vi "TeledyneVueCommand.vi"(4 "Channel Name":string="TeleVue:Mdot:Meas(g/min)", 6 "Port Name":string="tcp://192.168.124.71:10001", 7 "Timeout/ms":u32=1500, 8 "Numeric Value":dbl format="%.6g", 9 "TeledyneVueCommand":T2="FullScaleRatingSLPM", 10 "Address":u8=186 format="%.0x") -> (0 "String Reply":string="!11,100.0000\r\n", 1 "Error Description":string, 2 "Numeric Reply":dbl=100.0 format="%_6g", 3 "OK":bool)   [LabVIEW 2017]
uses:
  TeledyneVueCommand.ctl
  TeledyneDFCCommandDescriptor.ctl
  TeledyneVueCommandPhases.ctl
panel:
  out "commandString":string
  out "Audit trail":string[](array[string])
  out "CommandDescriptorOutput":T1={"Command"="FullScaleRatingSLPM", "Mnemonic"="E", "Min"=nan, "Max"=nan, "ActionPath"=["PassCommand", "Communicate", "ParseNumber", "Done"]}
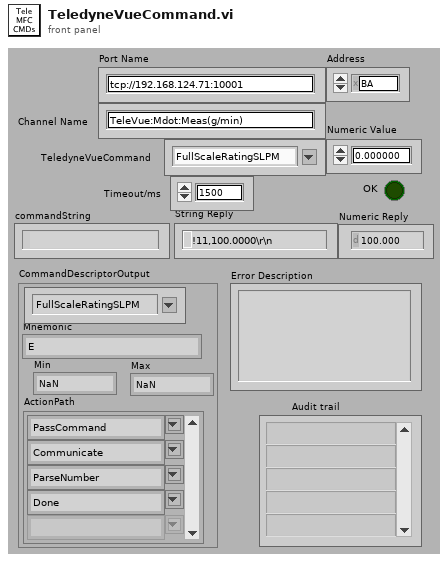
[diagram p1: front panel]
types:
  T1 = typedef "TeledyneDFCCommandDescriptor.ctl" = cluster{"Command":T2, "Mnemonic":string, "Min":dbl, "Max":dbl, "ActionPath":T3[]}
  T2 = typedef "TeledyneVueCommand.ctl" = string
  T3 = typedef "TeledyneVueCommandPhases.ctl" = string
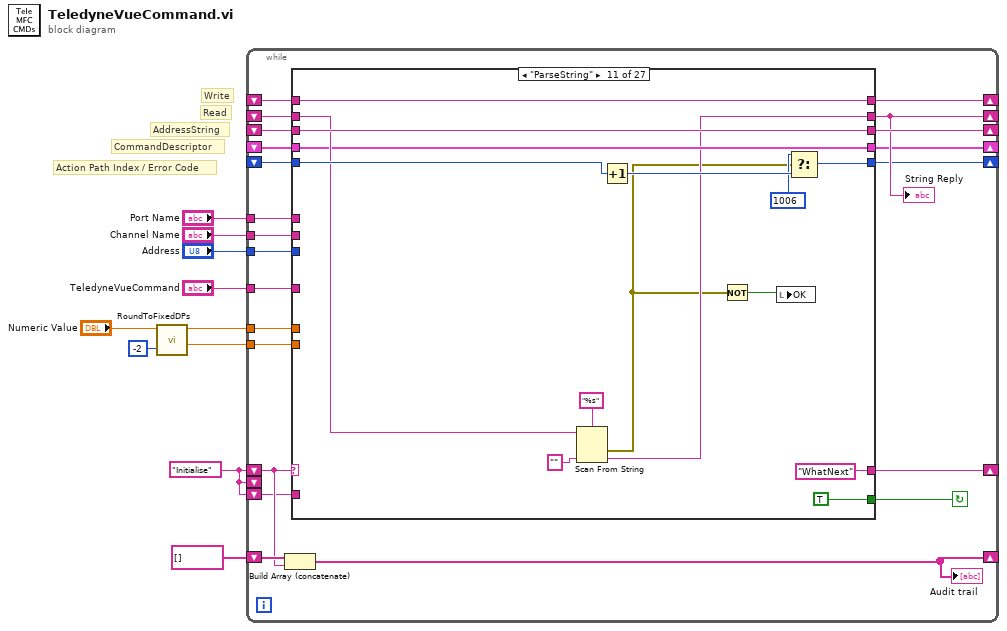
[diagram p0: block diagram]
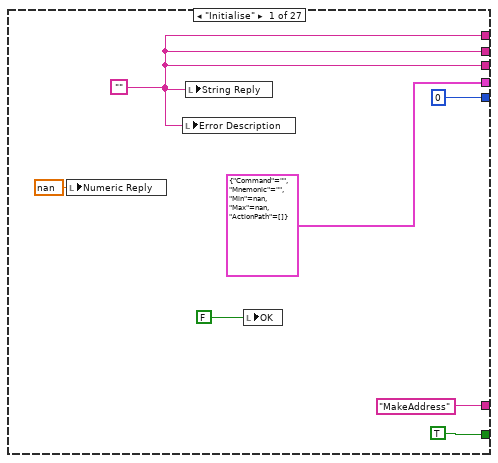
[diagram p2: hidden frame]
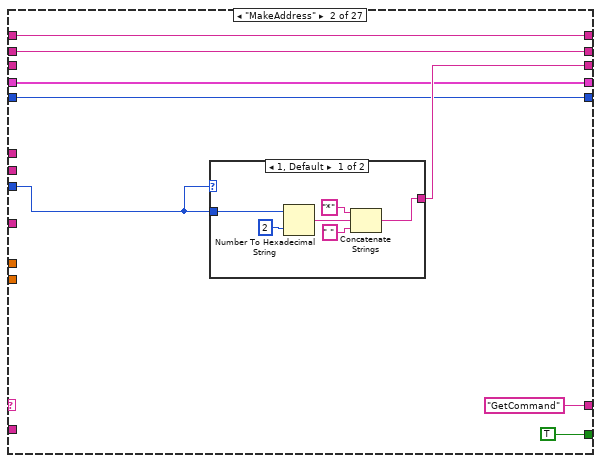
[diagram p3: hidden frame]
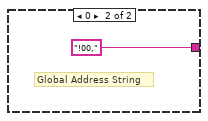
[diagram p4: hidden frame]
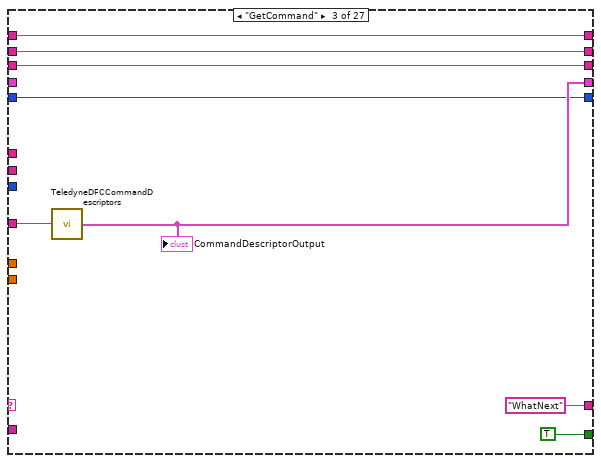
[diagram p5: hidden frame]
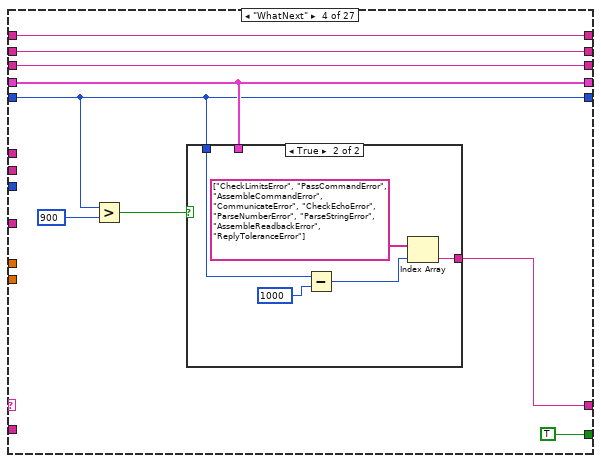
[diagram p6: hidden frame]
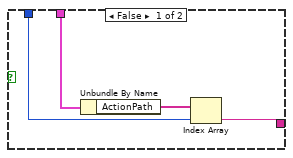
[diagram p7: hidden frame]
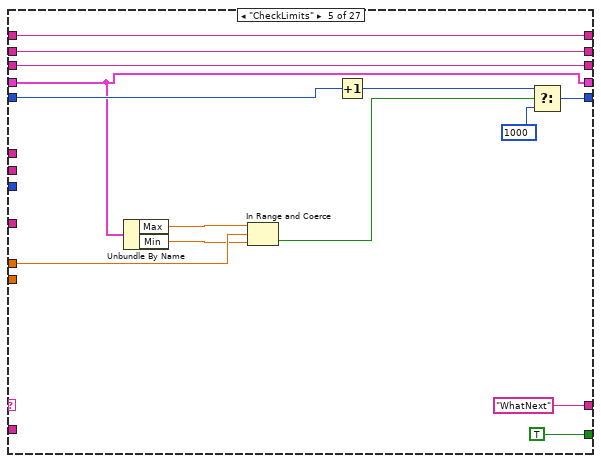
[diagram p8: hidden frame]
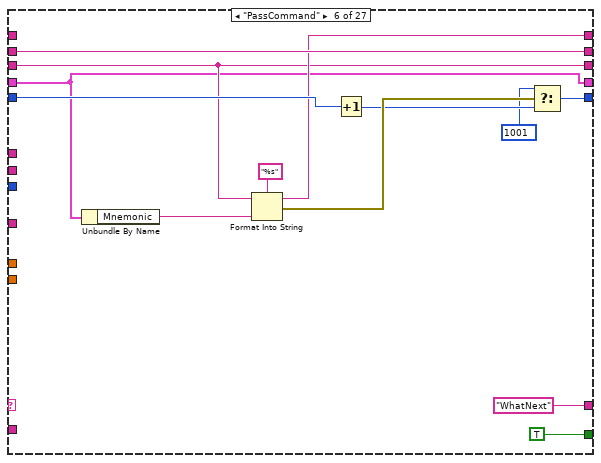
[diagram p9: hidden frame]
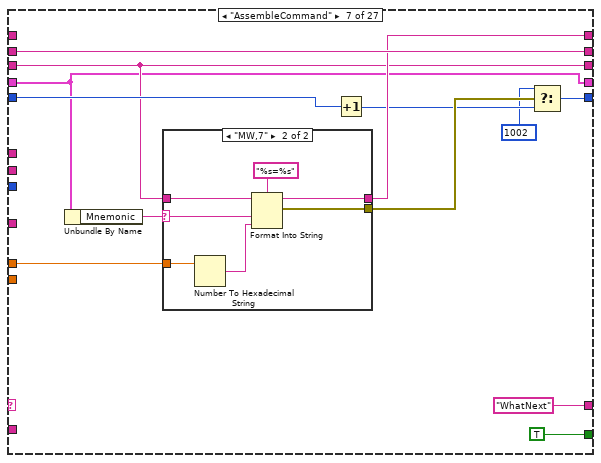
[diagram p10: hidden frame]
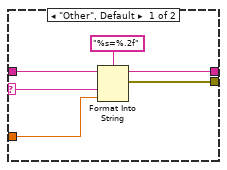
[diagram p11: hidden frame]
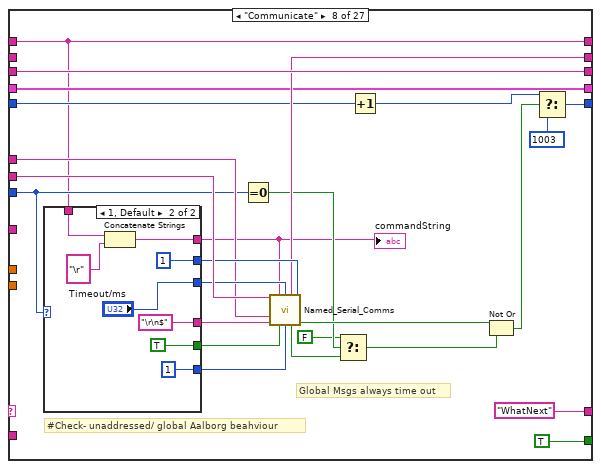
[diagram p12: hidden frame]
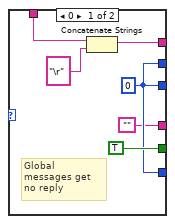
[diagram p13: hidden frame]
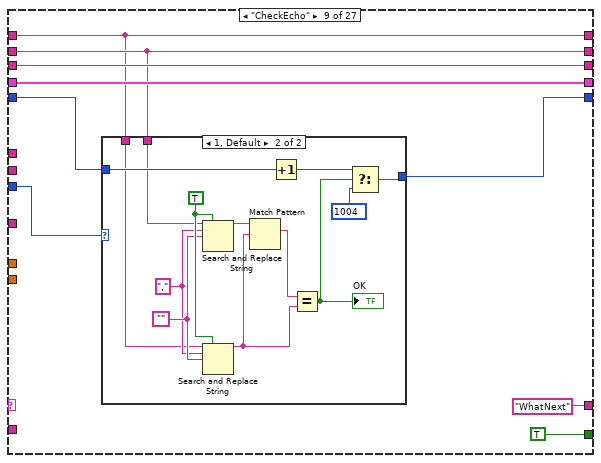
[diagram p14: hidden frame]
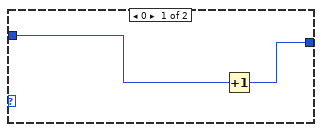
[diagram p15: hidden frame]
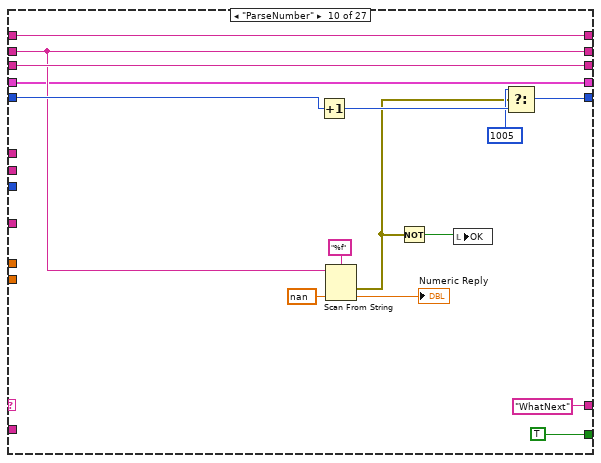
[diagram p16: hidden frame]
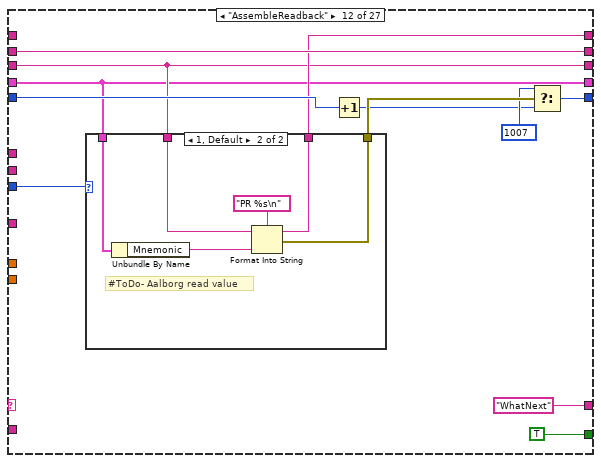
[diagram p17: hidden frame]
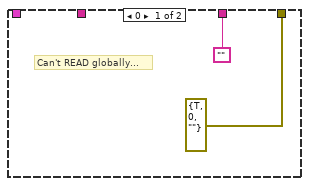
[diagram p18: hidden frame]
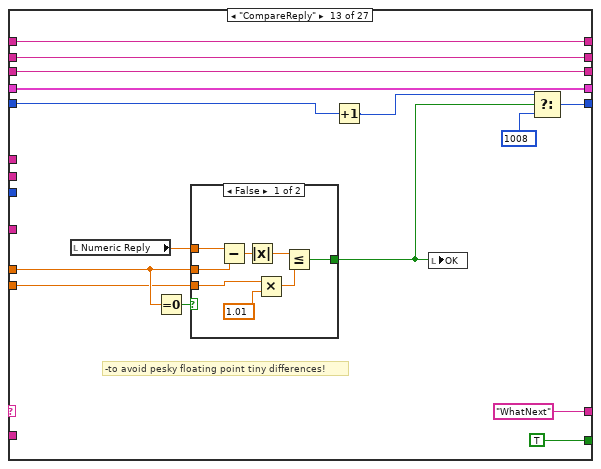
[diagram p19: hidden frame]
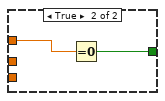
[diagram p20: hidden frame]
diagram:
  w5 = "Initialise"
  # "Action Path Index / Error Code"
  # "CommandDescriptor"
  # "AddressString"
  # "Read"
  # "Write"
  n1 = call "RoundToFixedDPs.vi"("Power of ten"=-2, "Number to round"="Numeric Value") -> ("Decimal place"=w1:dbl, "Rounded number"=w2:dbl)  [unwired: 8 in]
  n2 = while {
    shift-right: [w20] -> _
    shift-left: w5 -> [w14]
    tunnel: "Address" -> [w32]
    tunnel: "TeledyneVueCommand" -> [w31]
    tunnel: w2 -> [w30]
    shift-right: [w29] -> _
    shift-left: _ -> [w28]
    tunnel: "Port Name" -> [w27]
    tunnel: "Channel Name" -> [w26]
    shift-right: [w19] -> _
    shift-left: _ -> [w25]
    shift-right: [w23] -> _
    shift-left: _ -> [w22]
    shift-right: [w12] -> _
    shift-left: string[] [] -> [w21]
    shift-right: [w18] -> _
    shift-left: _ -> [w17]
    shift-right: [w15] -> _
    shift-left: _ -> [w16]
    shift-left: w5 -> [_]
    shift-left: w5 -> [w13]
    tunnel: w1 -> [w11]
    stop <- w24 continue-if-true
    n3 = Build Array (concatenate)(w21, w14) -> (w12:T3[])
    "Audit trail" <- w12
    n4 = case shown="\"ParseString\"" w14 {
      selector: w14 -> [_ _ _ _ _ _ _ _ _ _ _ _ _ _ _ _ _ _ _ _ _ _ _ _ _ _ w439]
      tunnel: ["MakeAddress" "GetCommand" "WhatNext" w67 "WhatNext" "WhatNext" "WhatNext" "WhatNext" "WhatNext" "WhatNext" "WhatNext" "WhatNext" "WhatNext" w275 "Error" "Initialise" "Error" "Error" "Error" "Error" "Error" "Error" "Error" "Error" "Error" "Error" w439] -> w20
      tunnel: w32 -> [_ w40 _ _ _ _ _ w136 w173 _ _ w230 _ _ _ _ w327 w338 w348 w359 w369 w382 w393 w404 w415 w424 _]
      tunnel: w31 -> [_ _ w59 _ _ _ _ _ _ _ _ _ _ _ _ _ _ _ _ _ _ _ _ _ _ _ _]
      tunnel: w30 -> [_ _ _ _ w92 _ w108 _ _ _ _ _ w248 _ _ _ w330 _ w351 _ _ _ _ _ _ _ _]
      tunnel: [w34 w45 w61 w70 w90 w102 w115 w135 w174 w203 w220 w233 w254 w281 w297 w309 w335 w345 w356 w366 w378 w390 w401 w412 w421 w432 w437] -> w29
      tunnel: w28 -> [_ w45 w61 w70 w90 _ _ w135 w174 w203 w220 _ w254 w281 w297 w319 _ _ _ _ w372 w384 _ _ _ _ _]
      tunnel: w27 -> [_ _ _ _ _ _ _ w152 _ _ _ _ _ _ _ w320 _ _ _ _ _ _ _ _ _ _ _]
      tunnel: w26 -> [_ _ _ _ _ _ _ w158 _ _ _ _ _ _ w292 w321 _ _ _ _ _ _ _ _ _ _ _]
      tunnel: [w34 w44 w60 w69 w94 w107 w120 w149 w175 w201 w215 w238 w261 w279 w302 w310 w335 w345 w356 w366 w378 w381 w401 w412 w421 w432 w437] -> w19
      tunnel: w25 -> [_ w44 w60 w69 w94 w107 w120 _ w175 w201 w218 w238 w261 w279 w302 w310 _ _ _ _ w371 w381 w395 w406 _ w426 _]
      tunnel: [TRUE TRUE ("Continue") TRUE ("Continue") TRUE ("Continue") TRUE TRUE TRUE TRUE TRUE TRUE TRUE TRUE TRUE w276 TRUE w311 TRUE ("Continue") TRUE ("Continue") TRUE ("Continue") TRUE ("Continue") TRUE ("Continue") TRUE ("Continue") TRUE ("Continue") TRUE ("Continue") TRUE ("Continue") TRUE ("Continue") FALSE] -> w24
      tunnel: [w34 w47 w58 w68 w93 w101 w114 w150 w180 w202 w219 w231 w256 w280 w307 w309 w335 w345 w356 w366 w378 w390 w401 w412 w421 w432 w437] -> w23
      tunnel: w22 -> [_ _ w58 w68 w93 w101 w114 w150 w180 w202 w219 w231 w256 w280 w307 _ _ _ _ _ _ _ _ _ _ _ _]
      tunnel: [T1 {"Command"="", "Mnemonic"="", "Min"=nan, "Max"=nan, "ActionPath"=[]} ("CommandDescriptorOutput") w42 w56 w66 w81 w98 w113 w148 w176 w200 w217 w229 w255 w273 w303 w325 w333 w343 w354 w364 w376 w388 w399 w410 w419 w430 w436] -> w18
      tunnel: w17 -> [_ w42 _ w66 w81 w98 w113 w148 w176 w200 w217 w229 w255 w272 w303 w325 w333 w343 w354 w364 w376 w388 w399 w410 w419 w430 w436]
      tunnel: w16 -> [_ w41 w55 w65 w85 w103 w116 w143 w177 w208 w223 w234 w257 _ w304 w324 w334 w344 w355 w365 w377 w389 w400 w411 w420 w431 w435]
      tunnel: [0 w41 w55 w65 w86 w104 w117 w145 w178 w209 w224 w235 w258 0 ("f") w305 w324 w334 w344 w355 w365 w377 w389 w400 w411 w420 w431 w435] -> w15
      tunnel: w13 -> [_ _ _ _ _ _ _ _ _ _ _ _ _ _ _ w317 _ _ _ _ _ _ _ _ _ _ _]
      tunnel: w11 -> [_ _ _ _ _ _ _ _ _ _ _ _ w247 _ _ _ _ _ _ _ _ _ _ _ _ _ _]
      frame "Initialise" {
        w34 = ""
        n5 = local write "Numeric Reply"(nan ("Numeric Reply")) -> ()
        n6 = local write "Error Description"(w34) -> ()
        n7 = local write "String Reply"(w34) -> ()
        n8 = local write "OK"(FALSE ("GoodEcho")) -> ()
      }
      frame "MakeAddress" {
        n9 = case shown="1, Default" w40 {
          tunnel: w40 -> [w48 _]
          tunnel: [w49 "!00,"] -> w47
          frame 1, Default {
            n10 = Number To Hexadecimal String(1:i16 2 ("width (-)"), 2:w48) -> (0:w52:string)
            n11 = Concatenate Strings("*" ("string"), w52, " " ("string")) -> (w49:string)
          }
          frame 0 {
            # "Global Address String"
          }
        }
      }
      frame "GetCommand" {
        n12 = call "TeledyneDFCCommandDescriptors.vi"("AalborgDFCCommand"=w59) -> ("CommandDescriptorOutput"=w56:T1)  [unwired: 4 out]
        "CommandDescriptorOutput" <- w56
      }
      frame "WhatNext" {
        n13 = Greater?(x=w65, y=900) -> (0:w63:bool)
        n14 = case shown="True" w63 {
          tunnel: [w74 w76] -> w67
          tunnel: w66 -> [w73 _]
          tunnel: w65 -> [w72 w79]
          frame False {
            n15 = Unbundle By Name(w73) -> ("ActionPath"=w75:T3[])
            n16 = Index Array(array=w75, index=w72) -> (element=w74:T3)
          }
          frame True {
            n17 = Subtract(x=w79, y=1000) -> (x-y=w77:i32)
            n18 = Index Array(array=string[] ["CheckLimitsError", "PassCommandError", "AssembleCommandError", "CommunicateError", "CheckEchoError", "ParseNumberError", "ParseStringError", "AssembleReadbackError", "ReplyToleranceError"], index=w77) -> (element=w76:string)
          }
        }
      }
      frame "CheckLimits" {
        n19 = Unbundle By Name(w81) -> ("Max"=w89:dbl, "Min"=w88:dbl)
        n20 = In Range and Coerce(upper limit=w89, x=w92, lower limit=w88) -> (In Range?=w83:bool)  [unwired: 1 out]
        n21 = Increment(x=w85) -> (x+1=w84:i32)
        n22 = Select(t=w84, s=w83, f=1000) -> (s? t:f=w86:i32)
      }
      frame "PassCommand" {
        n23 = Unbundle By Name(w98) -> ("Mnemonic"=w100:string)
        n24 = Format Into String(format string="%s", initial string=w101, w100) -> (resulting string=w102:string, error out=w97:errorcluster)  [unwired: 1 in]
        n25 = Increment(x=w103) -> (x+1=w96:i32)
        n26 = Select(t=1001 ("f"), s=w97, f=w96) -> (s? t:f=w104:i32)
      }
      frame "AssembleCommand" {
        n27 = Unbundle By Name(w113) -> ("Mnemonic"=w109:string)
        n28 = case shown="\"MW,7\"" w109 {
          selector: w109 -> [w121 w127]
          tunnel: [w126 w133] -> w115
          tunnel: w114 -> [w125 w132]
          tunnel: [w123 w130] -> w112
          tunnel: w108 -> [w122 w129]
          frame "Other", Default {
            n29 = Format Into String(format string="%s=%.2f", initial string=w125, w121, w122) -> (resulting string=w126:string, error out=w123:errorcluster)  [unwired: 1 in]
          }
          frame "MW,7" {
            n30 = Number To Hexadecimal String(2:w129) -> (0:w128:string)  [unwired: 1 in]
            n31 = Format Into String(format string="%s=%s", initial string=w132, w127, w128) -> (resulting string=w133:string, error out=w130:errorcluster)  [unwired: 1 in]
          }
        }
        n32 = Increment(x=w116) -> (x+1=w111:i32)
        n33 = Select(t=1002 ("f"), s=w112, f=w111) -> (s? t:f=w117:i32)
      }
      frame "Communicate" {
        # "#Check- unaddressed/ global Aalborg beahviour"
        # "Global Msgs always time out"
        n34 = case shown="1, Default" w136 {
          tunnel: ["" "\r\n$"] -> w157
          tunnel: [w163 1 ("Terminate Count")] -> w156
          tunnel: [w163 "Timeout/ms"] -> w155
          tunnel: [TRUE ("Log Errors?") TRUE ("Log Errors?")] -> w154
          tunnel: [w163 1 ("!Error retries")] -> w153
          tunnel: w135 -> [w160 w167]
          tunnel: [w161 w166] -> w134
          frame 0 {
            w163 = 0 ("!Error retries")
            # "Global messages get no reply"
            n35 = Concatenate Strings(w160, "\r" ("string")) -> (w161:string)
          }
          frame 1, Default {
            n36 = Concatenate Strings(w167, "\r" ("string")) -> (w166:string)
          }
        }
        "commandString" <- w134
        n37 = Equal To 0?(x=w136) -> (x = 0?=w139:bool)
        n38 = call "Named_Serial_Comms.vi"("Channel Name"=w158, "Write"=w134, "Timeout/ms"=w155, "!Error retries"=w153, "Port Name"=w152, "Term Grep"=w157, "Log Errors?"=w154, "Terminate Count"=w156) -> ("Read"=w149:string, "Timed out"=w138:bool, "Serial Error"=w146:bool)  [unwired: 1 in, 4 out]
        n39 = Select(t=FALSE, s=w139, f=w138) -> (s? t:f=w140:bool)
        n40 = Increment(x=w143) -> (x+1=w142:i32)
        n41 = Not Or(1:w140, 2:w146) -> (0:w144:bool)
        n42 = Select(t=w142, s=w144, f=1003) -> (s? t:f=w145:i32)
      }
      frame "CheckEcho" {
        n43 = case shown="1, Default" w173 {
          tunnel: [w182 w195] -> w178
          tunnel: w177 -> [w183 w193]
          tunnel: w175 -> [_ w186]
          tunnel: w174 -> [_ w185]
          frame 0 {
            n44 = Increment(x=w183) -> (x+1=w182:i32)
          }
          frame 1, Default {
            w187 = "," ("search string")
            w192 = TRUE ("replace all? (F)")
            w191 = ""
            n45 = Search and Replace String(replace all?=w192, input string=w186, search string=w187, replace string=w191) -> (result string=w190:string)  [unwired: 4 in, 3 out]
            n46 = Search and Replace String(replace all?=w192, input string=w185, search string=w187, replace string=w191) -> (result string=w188:string)  [unwired: 4 in, 3 out]
            n47 = Match Pattern(string=w190, regular expression=w188) -> (match substring=w189:string)  [unwired: 1 in, 3 out]
            n48 = Increment(x=w193) -> (x+1=w194:i32)
            n49 = Equal?(x=w189, y=w188) -> (x = y?=w184:bool)
            "OK" <- w184
            n50 = Select(t=w194, s=w184, f=1004) -> (s? t:f=w195:i32)
          }
        }
      }
      frame "ParseNumber" {
        n51 = Increment(x=w208) -> (x+1=w206:i32)
        n52 = Scan From String(format string="%f", input string=w201, default 1=nan ("default value 1")) -> (error out=w199:errorcluster, output 1=→"Numeric Reply":dbl)  [unwired: 2 in, 2 out]
        n53 = Not(x=w199) -> (.not. x?=w198:bool)
        n54 = local write "OK"(w198) -> ()
        n55 = Select(t=1005, s=w199, f=w206) -> (s? t:f=w209:i32)
      }
      frame "ParseString" {
        n56 = Scan From String(format string="%s", input string=w218, default 1="") -> (error out=w213:errorcluster, output 1=w215:string)  [unwired: 2 in, 2 out]
        n57 = Increment(x=w223) -> (x+1=w222:i32)
        n58 = Not(x=w213) -> (.not. x?=w214:bool)
        n59 = local write "OK"(w214) -> ()
        n60 = Select(t=1006, s=w213, f=w222) -> (s? t:f=w224:i32)
      }
      frame "AssembleReadback" {
        n61 = case shown="1, Default" w230 {
          tunnel: w229 -> [_ w246]
          tunnel: ["" w245] -> w233
          tunnel: [errorcluster {"status"=TRUE, "code"=0, "source"=""} ("error IO") w244] -> w232
          tunnel: w231 -> [_ w243]
          frame 0 {
            # "Can't READ globally..."
          }
          frame 1, Default {
            # "#ToDo- Aalborg read value"
            n62 = Unbundle By Name(w246) -> ("Mnemonic"=w242:string)
            n63 = Format Into String(format string="PR %s\n", initial string=w243, w242) -> (resulting string=w245:string, error out=w244:errorcluster)  [unwired: 1 in]
          }
        }
        n64 = Increment(x=w234) -> (x+1=w227:i32)
        n65 = Select(t=1007 ("f"), s=w232, f=w227) -> (s? t:f=w235:i32)
      }
      frame "CompareReply" {
        # "-to avoid pesky floating point tiny differences!"
        n66 = local read "Numeric Reply"() -> (w253:dbl)
        n67 = Equal To 0?(x=w248) -> (x = 0?=w249:bool)
        n68 = case shown="False" w249 {
          tunnel: w253 -> [w269 w271]
          tunnel: w248 -> [w267 _]
          tunnel: [w265 w270] -> w250
          tunnel: w247 -> [w263 _]
          frame False {
            n69 = Subtract(x=w269, y=w267) -> (x-y=w268:dbl)
            n70 = Absolute Value(x=w268) -> (abs(x)=w266:dbl)
            n71 = Multiply(x=w263, y=1.01) -> (x*y=w264:dbl)
            n72 = Less Or Equal?(x=w266, y=w264) -> (x <= y?=w265:bool)
          }
          frame True {
            n73 = Equal To 0?(x=w271) -> (x = 0?=w270:bool)
          }
        }
        n74 = Increment(x=w257) -> (x+1=w251:i32)
        n75 = local write "OK"(w250) -> ()
        n76 = Select(t=w251, s=w250, f=1008) -> (s? t:f=w258:i32)
      }
      frame "Done" {
        # "#Check- What is the error prompt from Aalborgs?"
        n77 = Match Pattern(string=w279, regular expression="?") -> (offset past match=w274:i32)  [unwired: 4 out]
        n78 = case shown="0, Default" w274 {
          tunnel: [TRUE ("Continue") FALSE ("Continue")] -> w276
          tunnel: ["WhatNext" "Initialise"] -> w275
          tunnel: [w285 w286] -> w273
          tunnel: w272 -> [_ w286]
          frame 0, Default {
            # "#Check- What should we do \nif there's an error?"
            n79 = call "TeledyneDFCCommandDescriptors.vi"("AalborgDFCCommand"=T2 "ValveStatus") -> ("CommandDescriptorOutput"=w285:T1)  [unwired: 4 out]
          }
          frame -1 {
          }
        }
      }
      frame "ParseError" {
        n80 = call <vilib>:"Trim Whitespace.vi"("string"=w297) -> ("trimmed string"=w295:string)  [unwired: 1 in]
        n81 = Concatenate Strings(w295, "%s" ("format string")) -> (w298:string)
        n82 = Scan From String(format string=w298, input string=w302, default 1="") -> (error out=w301:errorcluster, output 1=w293:string)  [unwired: 2 in, 2 out]
        n83 = call "TeledyneVueErrorCodes.vi"("Error Code"=w293) -> ("Error Description"=w291:string)  [unwired: 4 out]
        n84 = Increment(x=w304) -> (x+1=w300:i32)
        n85 = Format Into String(format string="The %s has %s", w292, w291) -> (resulting string=→"Error Description":string)  [unwired: 2 in, 1 out]
        n86 = Select(t=1007, s=w301, f=w300) -> (s? t:f=w305:i32)
      }
      frame "Error" {
        w314 = "Error in AalborgDFCCommand.vi: " ("string")
        w309 = ""
        w311 = FALSE ("Continue")
        n87 = local read "Error Description"() -> (w313:string)
        n88 = call "Serial_log_build.vi"("Read"=w310, "Write String"=w319, "Port Name"=w320) -> ("Output Array"=w322:string[])
        n89 = Empty String/Path?(string/path=w313) -> (empty?=w318:bool)
        n90 = Concatenate Strings(w314, w317) -> (w316:string)
        n91 = Concatenate Strings(w314, w313) -> (w315:string)
        n92 = Select(t=w316, s=w318, f=w315) -> (s? t:f=w312:string)
        n93 = call "Write_serial_log.vi"("Log Type"="AalborgDFC_Error_Log", "Log Array"=w322, "Header message"=w312, "Channel Name"=w321) -> ()  [unwired: 1 out]
        n94 = local write "OK"(w311) -> ()
      }
      frame "CheckLimitsError" {
        w335 = ""
        n95 = Unbundle By Name(w333) -> ("Mnemonic"=w331:string)
        n96 = Format Into String(format string="%s=%d) to MFC %x", initial string="Attempt to Write an out-of-range value (" ("message"), w331, w330, w327) -> (resulting string=w328:string)  [unwired: 1 in, 1 out]
        n97 = local write "Error Description"(w328) -> ()
      }
      frame "PassCommandError" {
        w345 = ""
        n98 = Unbundle By Name(w343) -> ("Mnemonic"=w341:string)
        n99 = Format Into String(format string="%s) to MFC %x", initial string="Attempt to PassCommand (" ("message"), w341, w338) -> (resulting string=w339:string)  [unwired: 1 in, 1 out]
        n100 = local write "Error Description"(w339) -> ()
      }
      frame "AssembleCommandError" {
        w356 = ""
        n101 = Unbundle By Name(w354) -> ("Mnemonic"=w352:string)
        n102 = Format Into String(format string="%s,%.1f) to MFC %x", initial string="Attempt to AssembleCommand (" ("message"), w352, w351, w348) -> (resulting string=w349:string)  [unwired: 1 in, 1 out]
        n103 = local write "Error Description"(w349) -> ()
      }
      frame "CommunicateError" {
        w366 = ""
        n104 = Unbundle By Name(w364) -> ("Command"=w362:T2)
        n105 = Format Into String(format string="%s) to MFC %x", initial string="Serial CommsError (" ("message"), w362, w359) -> (resulting string=w360:string)  [unwired: 1 in, 1 out]
        n106 = local write "Error Description"(w360) -> ()
      }
      frame "CheckEchoError" {
        w378 = ""
        n107 = Unbundle By Name(w376) -> ("Command"=w374:T2)
        n108 = Format Into String(format string="Command = %s; Write = %s; Read=%s) to MFC %x", initial string="Echo Error (" ("message"), w374, w372, w371, w369) -> (resulting string=w370:string)  [unwired: 1 in, 1 out]
        n109 = local write "Error Description"(w370) -> ()
      }
      frame "ReplyToleranceError" {
        w390 = ""
        n110 = Unbundle By Name(w388) -> ("Command"=w386:T2)
        n111 = Format Into String(format string="Command = %s; Write = %s; Read=%s) to MFC %x", initial string="Reply out of tolerance (" ("message"), w386, w384, w381, w382) -> (resulting string=w383:string)  [unwired: 1 in, 1 out]
        n112 = local write "Error Description"(w383) -> ()
      }
      frame "ParseNumberError" {
        w401 = ""
        n113 = Unbundle By Name(w399) -> ("Mnemonic"=w397:string)
        n114 = Format Into String(format string="%s=%s) from MFC %x", initial string="Attempt to ParseNumber (" ("message"), w397, w395, w393) -> (resulting string=w394:string)  [unwired: 1 in, 1 out]
        n115 = local write "Error Description"(w394) -> ()
      }
      frame "ParseStringError" {
        w412 = ""
        n116 = Unbundle By Name(w410) -> ("Mnemonic"=w408:string)
        n117 = Format Into String(format string="%s=%s) from MFC %x", initial string="Attempt to ParseString (" ("message"), w408, w406, w404) -> (resulting string=w405:string)  [unwired: 1 in, 1 out]
        n118 = local write "Error Description"(w405) -> ()
      }
      frame "AssembleReadbackError" {
        w421 = ""
        n119 = Format Into String(format string="to MFC %x", initial string="Attempt to AssembleReadback " ("message"), w415) -> (resulting string=w416:string)  [unwired: 1 in, 1 out]
        n120 = local write "Error Description"(w416) -> ()
      }
      frame "ParseErrorError" {
        w432 = ""
        n121 = Unbundle By Name(w430) -> ("Command"=w428:T2)
        n122 = Format Into String(format string="Command = %s; Read = %s) for MFC %x", initial string="Attempt to ParseError (" ("message"), w428, w426, w424) -> (resulting string=w425:string)  [unwired: 1 in, 1 out]
        n123 = local write "Error Description"(w425) -> ()
      }
      frame "NoMatch", Default {
        w437 = ""
        n124 = One Button Dialog(message="Case not found in TeledyneDFCDriveCommand.vi", button name ("OK")="Shit!...") -> ()  [unwired: 1 out]
      }
    }
    "String Reply" <- w19
  }
